vi "Write Protocol ID.vi"(8 "error in (no error)":errorcluster, 10 "Protocol ID":u16, 11 "MB_ADU_TCP in":refnum<class "MB_ADU_TCP.lvclass">) -> (0 "error out":errorcluster, 3 "MB_ADU_TCP out":refnum<class "MB_ADU_TCP.lvclass">)   [LabVIEW 2016, in "MB Master.lvlib" / "MB_ADU_TCP.lvclass"]
uses:
  MB_ADU_TCP.lvclass
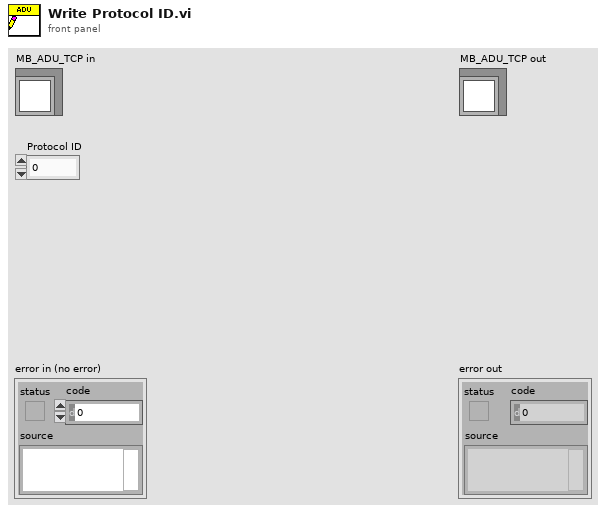
[diagram p1: front panel]
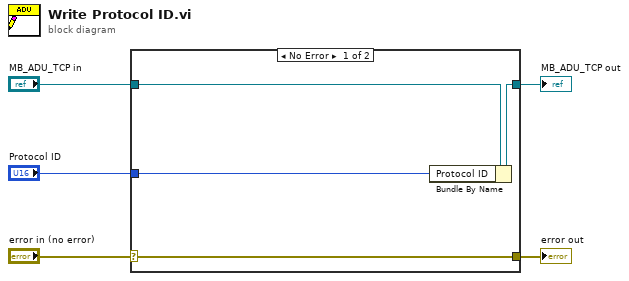
[diagram p0: block diagram]
diagram:
  n1 = case shown="No Error" "error in (no error)" {
    selector: "error in (no error)" -> [w9 w10]
    tunnel: [w9 w10] -> w4
    tunnel: [w7 w11] -> w2
    tunnel: "MB_ADU_TCP in" -> [w8 w11]
    tunnel: "Protocol ID" -> [w6 _]
    frame No Error {
      n2 = Bundle By Name(cluster=w8, "Protocol ID"=w6) -> (w7:refnum<class "MB_ADU_TCP.lvclass">)
    }
    frame Error {
    }
  }
  "error out" <- w4
  "MB_ADU_TCP out" <- w2
